vi "Write Output Conversion.vi"(9 "Process Data Output":u8[](array[numeric]), 10 "Map IN":map{string, dbl}(c390), 11 "Drives":T1(array[cluster])) -> (3 "Map OUT":map{string, dbl}(c390))   [LabVIEW 2024, in "EtherCAT Model.lvlib"]
uses:
  EtherCAT Model.lvlib
  <instrlib>/_Ackermann Automation/EtherCAT Lib/EcatLib/EthercatLib.lvlib
  <instrlib>/_Ackermann Automation/EtherCAT Lib/EcatLib/Conversion/ConvertFrameToBoolean.vi
  <instrlib>/_Ackermann Automation/EtherCAT Lib/EcatLib/Conversion/ConvertFrameToU16.vi
  <instrlib>/_Ackermann Automation/EtherCAT Lib/EcatLib/Conversion/ConvertFrameToI16.vi
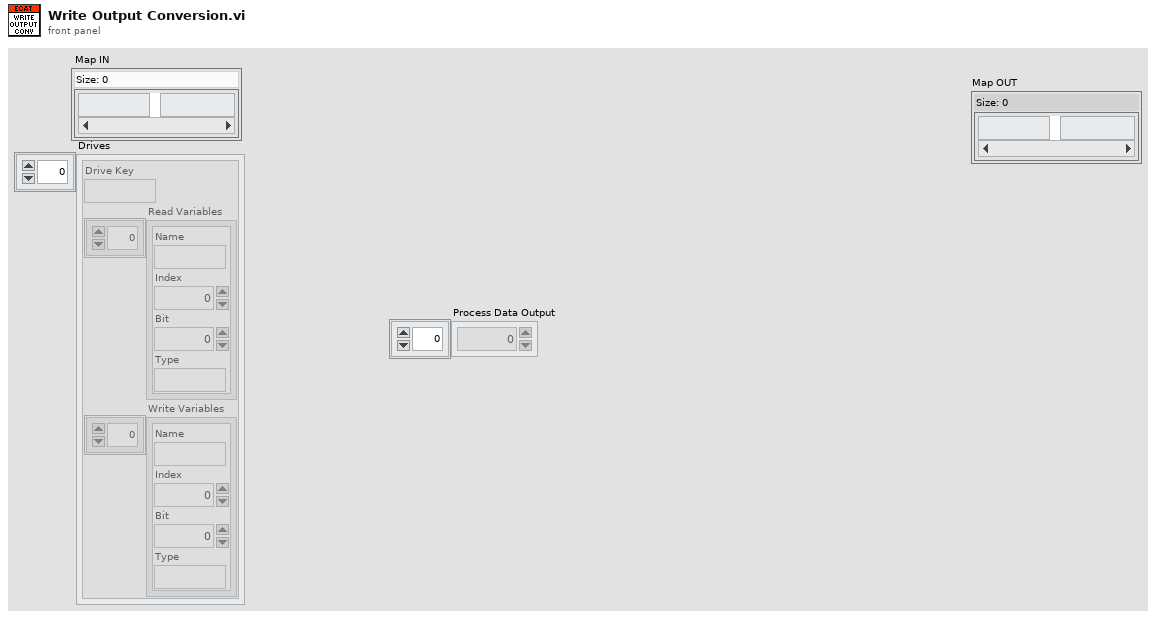
[diagram p1: front panel]
types:
  T1 = cluster{"Drive Key":string, "Read Variables":cluster{"Name":string, "Index":i32, "Bit":u8, "Type":string}[], "Write Variables":cluster{"Name":string, "Index":i32, "Bit":u8, "Type":string}[]}[]
  T2 = cluster{"Name":string, "Index":i32, "Bit":u8, "Type":string}[]
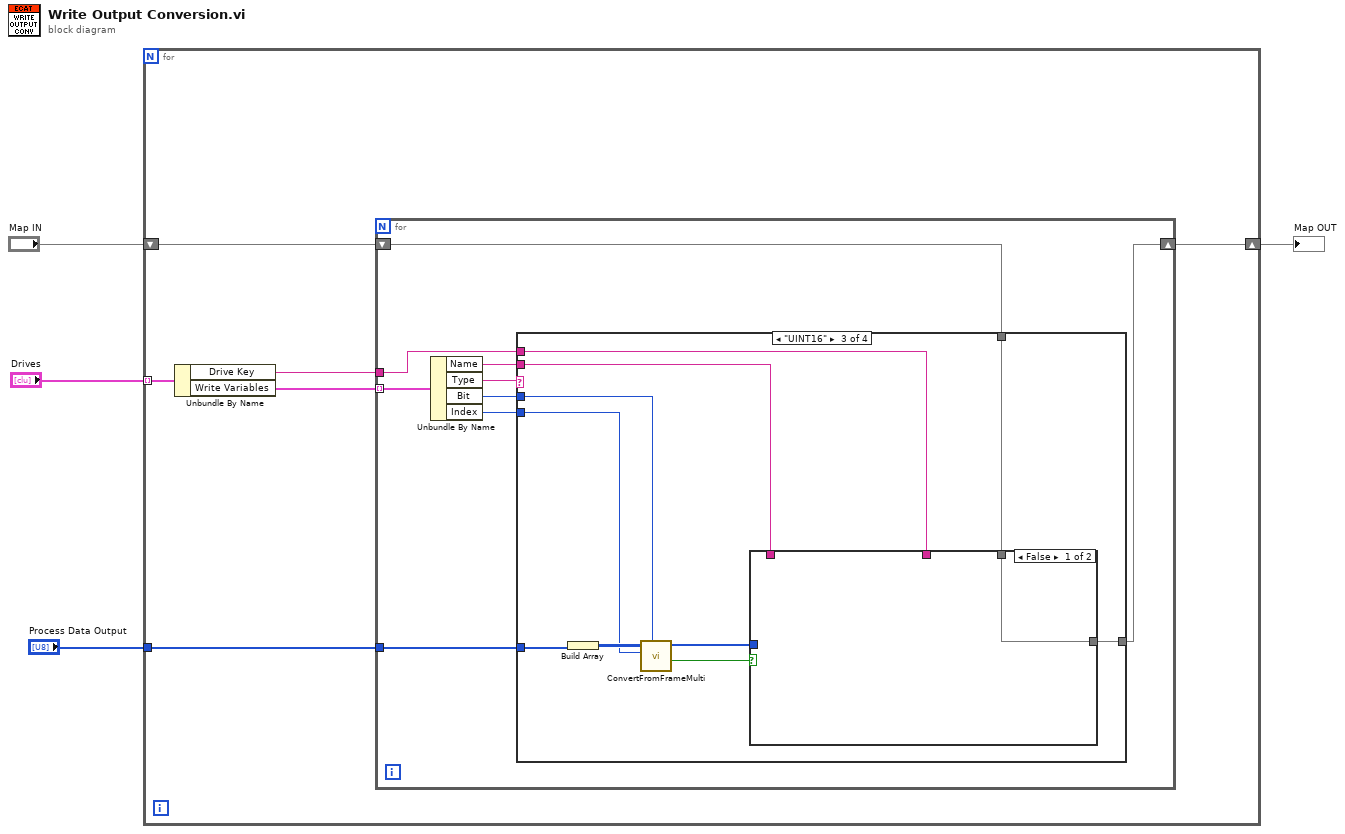
[diagram p0: block diagram]
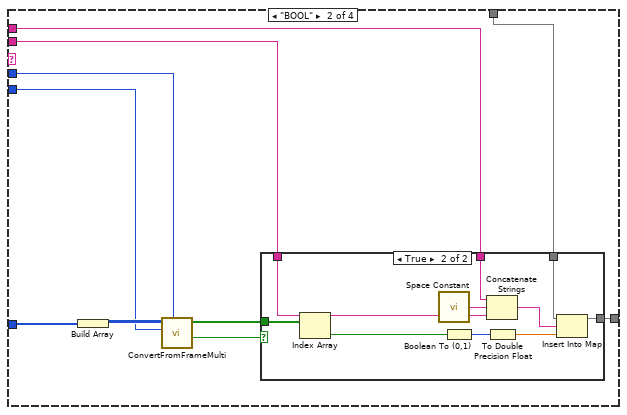
[diagram p3: hidden frame]
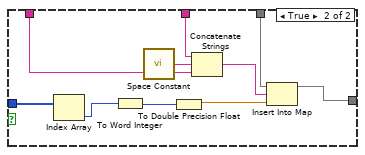
[diagram p5: hidden frame]
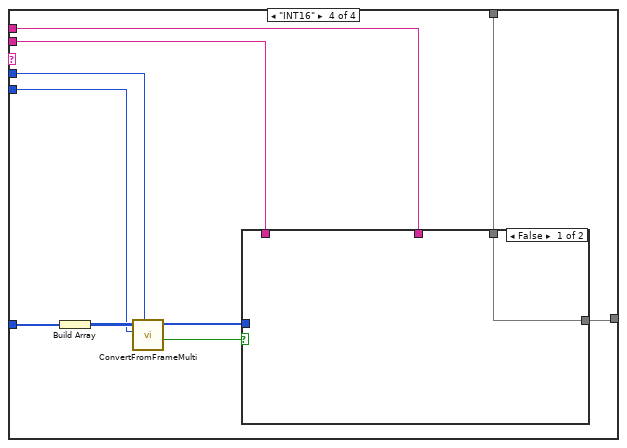
[diagram p6: hidden frame]
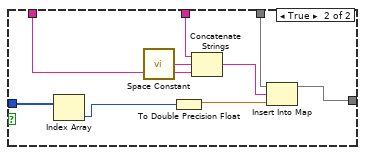
[diagram p7: hidden frame]
diagram:
  n1 = for {
    tunnel: "Drives" -> [w10] mode=indexing
    shift-right: [w5] -> w1
    shift-left: "Map IN" -> [w8]
    tunnel: "Process Data Output" -> [w6]
    n2 = Unbundle By Name(w10) -> ("Drive Key"=w7:string, "Write Variables"=w9:T2)
    n3 = for {
      tunnel: w9 -> [w19] mode=indexing
      shift-right: [w11] -> w5
      shift-left: w8 -> [w12]
      tunnel: w7 -> [w13]
      tunnel: w6 -> [w17]
      n4 = Unbundle By Name(w19) -> ("Name"=w14:string, "Type"=w18:string, "Bit"=w16:u8, "Index"=w15:i32)
      n5 = case shown="\"UINT16\"" w18 {
        tunnel: [w20 w28 w50 w70] -> w11
        tunnel: w17 -> [_ w25 w48 w69]
        tunnel: w16 -> [_ w27 w45 w67]
        tunnel: w15 -> [_ w24 w46 w66]
        tunnel: w14 -> [_ w23 w44 w65]
        tunnel: w13 -> [_ w22 w43 w64]
        tunnel: w12 -> [w20 w21 w42 w63]
        frame Default {
        }
        frame "BOOL" {
          n6 = Build Array(w25) -> (w26:u8[][])
          n7 = call-poly <instrlib>:"ConvertFromFrameMulti.vi"("Bit Index"=w27, "Byte Index"=w24, "Acquisition Data"=w26) -> ("Output Data Valid"=w30:bool, "Bit"=w29:bool[])  [unwired: 7 in]
          n8 = case shown="True" w30 {
            tunnel: w29 -> [_ w41]
            tunnel: [w31 w35] -> w28
            tunnel: w23 -> [_ w34]
            tunnel: w22 -> [_ w33]
            tunnel: w21 -> [w31 w32]
            frame False {
            }
            frame True {
              n9 = Index Array(array=w41) -> (element=w40:bool)  [unwired: 1 in]
              n10 = call <vilib>:"Space Constant.vi"() -> ("String"=w37:string)
              n11 = Boolean To (0,1)(Boolean=w40) -> (0, 1=w39:i16)
              n12 = Concatenate Strings(w33, w37, w34) -> (w36:string)
              n13 = To Double Precision Float(number=w39) -> (double precision float=w38:dbl)
              n14 = Insert Into Map(map in=w32, key=w36, value=w38) -> (map out=w35:map{string, dbl})  [unwired: 2 out]
            }
          }
        }
        frame "UINT16" {
          n15 = Build Array(w48) -> (w47:u8[][])
          n16 = call-poly <instrlib>:"ConvertFromFrameMulti.vi"("Bit Index"=w45, "Byte Index"=w46, "Acquisition Data"=w47) -> ("Output Data Valid"=w51:bool, "U16"=w49:u16[])  [unwired: 7 in]
          n17 = case shown="False" w51 {
            tunnel: [w52 w58] -> w50
            tunnel: w49 -> [_ w61]
            tunnel: w44 -> [_ w55]
            tunnel: w43 -> [_ w54]
            tunnel: w42 -> [w52 w53]
            frame False {
            }
            frame True {
              n18 = Index Array(array=w61) -> (element=w60:u16)  [unwired: 1 in]
              n19 = To Word Integer(number=w60) -> (16bit integer=w62:i16)
              n20 = call <vilib>:"Space Constant.vi"() -> ("String"=w57:string)
              n21 = To Double Precision Float(number=w62) -> (double precision float=w59:dbl)
              n22 = Concatenate Strings(w54, w57, w55) -> (w56:string)
              n23 = Insert Into Map(map in=w53, key=w56, value=w59) -> (map out=w58:map{string, dbl})  [unwired: 2 out]
            }
          }
        }
        frame "INT16" {
          n24 = Build Array(w69) -> (w68:u8[][])
          n25 = call-poly <instrlib>:"ConvertFromFrameMulti.vi"("Bit Index"=w67, "Byte Index"=w66, "Acquisition Data"=w68) -> ("Output Data Valid"=w72:bool, "I16"=w71:i16[])  [unwired: 7 in]
          n26 = case shown="False" w72 {
            tunnel: [w73 w79] -> w70
            tunnel: w71 -> [_ w82]
            tunnel: w65 -> [_ w76]
            tunnel: w64 -> [_ w75]
            tunnel: w63 -> [w73 w74]
            frame False {
            }
            frame True {
              n27 = Index Array(array=w82) -> (element=w81:i16)  [unwired: 1 in]
              n28 = call <vilib>:"Space Constant.vi"() -> ("String"=w78:string)
              n29 = To Double Precision Float(number=w81) -> (double precision float=w80:dbl)
              n30 = Concatenate Strings(w75, w78, w76) -> (w77:string)
              n31 = Insert Into Map(map in=w74, key=w77, value=w80) -> (map out=w79:map{string, dbl})  [unwired: 2 out]
            }
          }
        }
      }
    }
  }
  "Map OUT" <- w1
